vi "SetBackgroundImage.vi"(8 "error in (no error)":errorcluster caption="错误输入（无错误）", 10 "filename":string, 11 "StatusStripClass 输入":refnum<class "StatusStripClass.lvclass"> caption="DNL_LabVIEW Object in") -> (0 "error out":errorcluster caption="错误输出", 3 "StatusStripClass 输出":refnum<class "StatusStripClass.lvclass"> caption="DNL_LabVIEW Object out")   [LabVIEW 2013, in "StatusStripClass.lvclass"]
uses:
  StatusStripClass.lvclass
  StatusStripClass.lvclass/StatusStripClass.ctl
  System.Drawing
  System.Windows.Forms
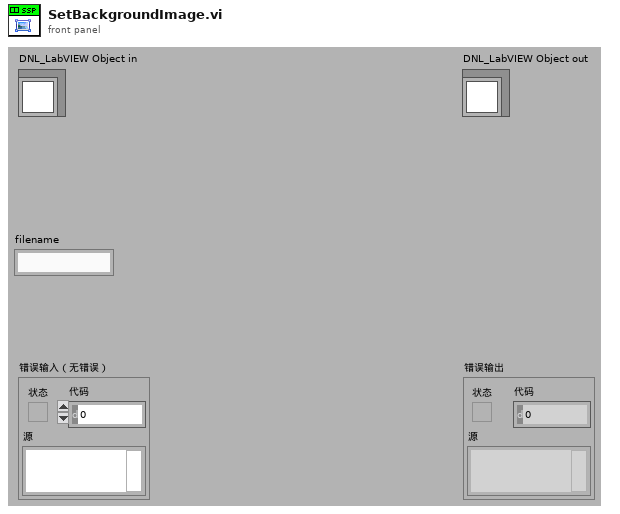
[diagram p1: front panel]
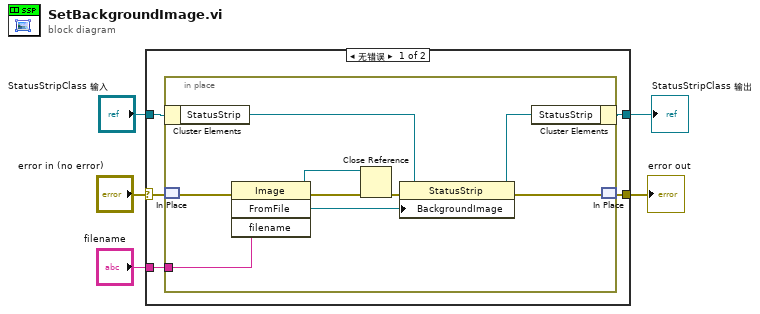
[diagram p0: block diagram]
diagram:
  n1 = case shown="无错误" "error in (no error)" {
    selector: "error in (no error)" -> [w8 w21]
    tunnel: [w7 w21] -> w4
    tunnel: [w6 w20] -> w2
    tunnel: "StatusStripClass 输入" -> [w9 w20]
    tunnel: "filename" -> [w10 _]
    frame No Error {
      n2 = in-place {
        in-place-border: w10 -> [w19]
        n3 = in-place-cluster #1(w9) -> ("StatusStrip"=w18:refnum<k24>)
        n4 = in-place-match #2(w8) -> (w14:errorcluster)
        n5 = invoke class="Image" method="FromFile"(error in=w14, "filename"=w19) -> (reference out=w15:refnum<k24>, error out=w13:errorcluster, "FromFile"=w16:refnum<k24>)  [unwired: 2 in, 1 out]
        n6 = Close Reference(reference=w15, error in (no error)=w13) -> (error out=w12:errorcluster)
        n7 = property class="StatusStrip"(reference=w18, error in=w12, "BackgroundImage"=w16) -> (reference out=w17:refnum<k24>, error out=w11:errorcluster)
        n8 = in-place-cluster #1("StatusStrip"=w17) -> (w6:refnum<class "StatusStripClass.lvclass">)
        n9 = in-place-match #2(w11) -> (w7:errorcluster)
      }
    }
    frame Error {
    }
  }
  "error out" <- w4
  "StatusStripClass 输出" <- w2
